vi "updata NodePath for traverse.vi"(8 "error in (no error)":errorcluster caption="错误输入（无错误）", 9 "Data in":string, 11 "Class in":refnum<class "PanelLinkNode.lvclass">) -> (0 "error out":errorcluster caption="错误输出", 1 "Data out":string, 3 "Class out":refnum<class "PanelLinkNode.lvclass"> caption="DNL_LabVIEW Object out")   [LabVIEW 2013, in "PanelLinkNode.lvclass"]
uses:
  PanelLinkNode.lvclass
  PanelObject/PanelObject.lvclass
  PanelLinkNode.lvclass/PanelLinkNode.ctl
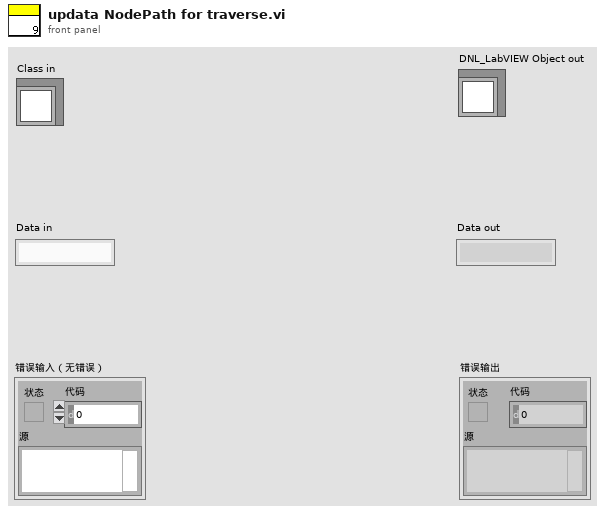
[diagram p1: front panel]
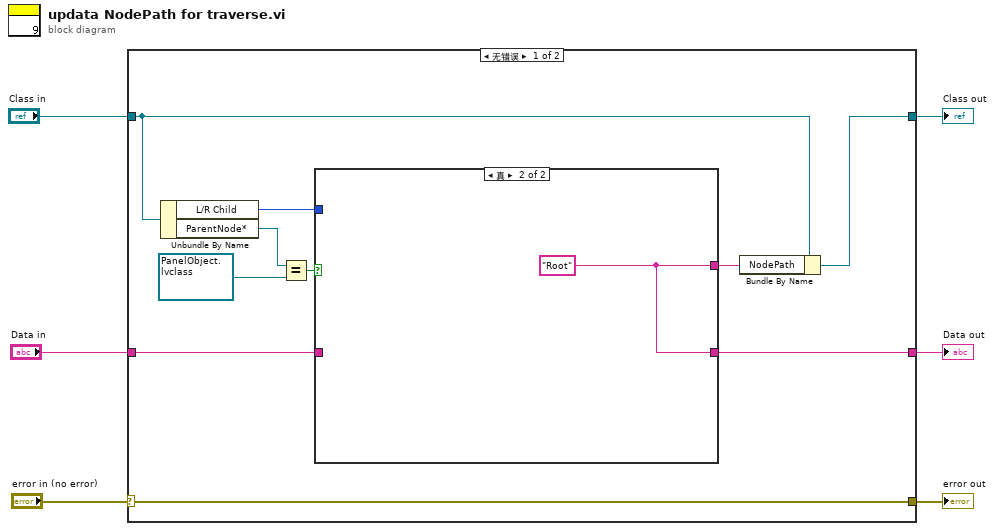
[diagram p0: block diagram]
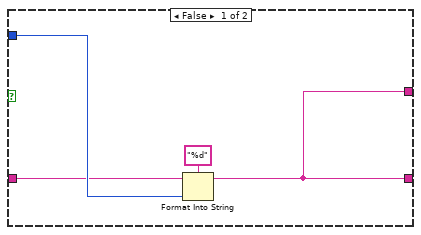
[diagram p2: hidden frame]
diagram:
  n1 = case shown="无错误" "error in (no error)" {
    selector: "error in (no error)" -> [w9 w24]
    tunnel: [w9 w24] -> w5
    tunnel: [w16 w23] -> w4
    tunnel: "Class in" -> [w10 w23]
    tunnel: "Data in" -> [w8 w22]
    tunnel: [w7 w22] -> w1
    frame No Error {
      n2 = Unbundle By Name(w10) -> ("L/R Child"=w12:u8, "ParentNode*"=w13:refnum<data-value>)
      n3 = Equal?(x=w13, y=refnum<data-value> refnum) -> (x = y?=w14:bool)
      n4 = case shown="真" w14 {
        tunnel: w12 -> [w19 _]
        tunnel: [w17 w21] -> w11
        tunnel: w8 -> [w18 _]
        tunnel: [w17 w21] -> w7
        frame False {
          n5 = Format Into String(format string="%d" ("格式字符串"), initial string=w18, w19) -> (resulting string=w17:string)  [unwired: 1 in, 1 out]
        }
        frame True {
          w21 = "Root"
        }
      }
      n6 = Bundle By Name(cluster=w10, "NodePath"=w11) -> (w16:refnum<class "PanelLinkNode.lvclass">)
    }
    frame Error {
    }
  }
  "error out" <- w5
  "Class out" <- w4
  "Data out" <- w1
